vi "Run.vi"(0 "reference in":refnum<class "Test3(BrRef).lvclass">, 5 "error in (no error)":errorcluster) -> (14 "reference out":refnum<class "Test3(BrRef).lvclass">, 19 "error out":errorcluster)   [LabVIEW 2016, in "Test3(BrRef).lvclass"]
uses:
  Test3(BrRef).lvclass
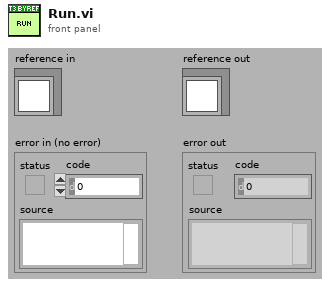
[diagram p1: front panel]
types:
  T1 = typedef "Test3(BrRef).lvclass/ObjectAttributes.ctl" = cluster{"Attribute1":dbl}
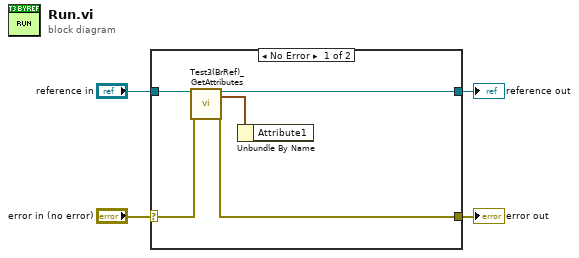
[diagram p0: block diagram]
diagram:
  n1 = case shown="No Error" "error in (no error)" {
    selector: "error in (no error)" -> [w9 w11]
    tunnel: [w7 w11] -> w3
    tunnel: [w5 w10] -> w1
    tunnel: "reference in" -> [w6 w10]
    frame No Error {
      n2 = call "Test3(BrRef)_GetAttributes.vi"("reference in"=w6, "error in (no error)"=w9) -> ("reference out"=w5:refnum<class "Test3(BrRef).lvclass">, "Data"=w8:T1, "error out"=w7:errorcluster)  [unwired: 14 in, 1 out]
      n3 = Unbundle By Name(w8) -> ()  [unwired: 1 out]
    }
    frame Error {
    }
  }
  "error out" <- w3
  "reference out" <- w1
